vi "Run.vi"(7 "Team Index":i32, 8 "Column":i32, 9 "Row":i32, 10 "View":i32[](array[numeric]) caption="View (Team Index, -1: empty)", 11 "Runner in":refnum<class "Finish.lvclass">) -> (0 "Replicated":refnum<class "Square.lvclass">, 1 "Direction":T1, 2 "Action":T2, 3 "Square Out":refnum<class "Square.lvclass">)   [LabVIEW 2015, in "Finish.lvclass"]
uses:
  Finish.lvclass
  Square/Square.lvclass
  Type Defs/Action Enum.ctl
  Type Defs/Direction Enum.ctl
  Common/Attack Options.ctl
  Common/Find Enemy.vi
  Common/Reverse Direction.vi
  Common/Common.lvlib
  Type Defs/SB Type Defs.lvlib
panel:
  # "NW\nN\nNE\nE\nSE\nS\nSW\nW"
  # "NOTICE - YOU MUST NOT REMOVE THIS NOTICE. PER THE FOLLOWING LICENSE, YOU MAY REPRODUCE THIS SOFTWARE PROVIDED YOU FOLLOW THE TERMS\nOF THE LICENSE.\n\n---BEGIN BSD LICENSE (http://opensource.org/licenses/BSD-2-Clause)---\nCopyright (c) 2015, Endigit, Inc. <robert@endigit.com>\nAll rights reserved.\n\nRedistribution and use in source and binary forms, with or without modification, are permitted provided that the following conditions are met:\n\n1. Redistributions of source code must retain the above copyright notice, this list of conditions and the following disclaimer.\n\n2. Redistributions in binary form must reproduce the above copyright notice, this list of conditions and the following disclaimer in the documentation and/or other \nmaterials provided with the distribution.\n\nTHIS SOFTWARE IS PROVIDED BY THE COPYRIGHT HOLDERS AND CONTRIBUTORS \"AS IS\" AND ANY EXPRESS OR IMPLIED WARRANTIES, INCLUDING, BUT NOT \nLIMITED TO, THE IMPLIED WARRANTIES OF MERCHANTABILITY AND FITNESS FOR A PARTICULAR PURPOSE ARE DISCLAIMED. IN NO EVENT SHALL THE COPYRIGHT \nHOLDER OR CONTRIBUTORS BE LIABLE FOR ANY DIRECT, INDIRECT, INCIDENTAL, SPECIAL, EXEMPLARY, OR CONSEQUENTIAL DAMAGES (INCLUDING, BUT NOT \nLIMITED TO, PROCUREMENT OF SUBSTITUTE GOODS OR SERVICES; LOSS OF USE, DATA, OR PROFITS; OR BUSINESS INTERRUPTION) HOWEVER CAUSED AND ON \nANY THEORY OF LIABILITY, WHETHER IN CONTRACT, STRICT LIABILITY, OR TORT (INCLUDING NEGLIGENCE OR OTHERWISE) ARISING IN ANY WAY OUT OF THE USE \nOF THIS SOFTWARE, EVEN IF ADVISED OF THE POSSIBILITY OF SUCH DAMAGE.\n---END BSD LICENSE---"
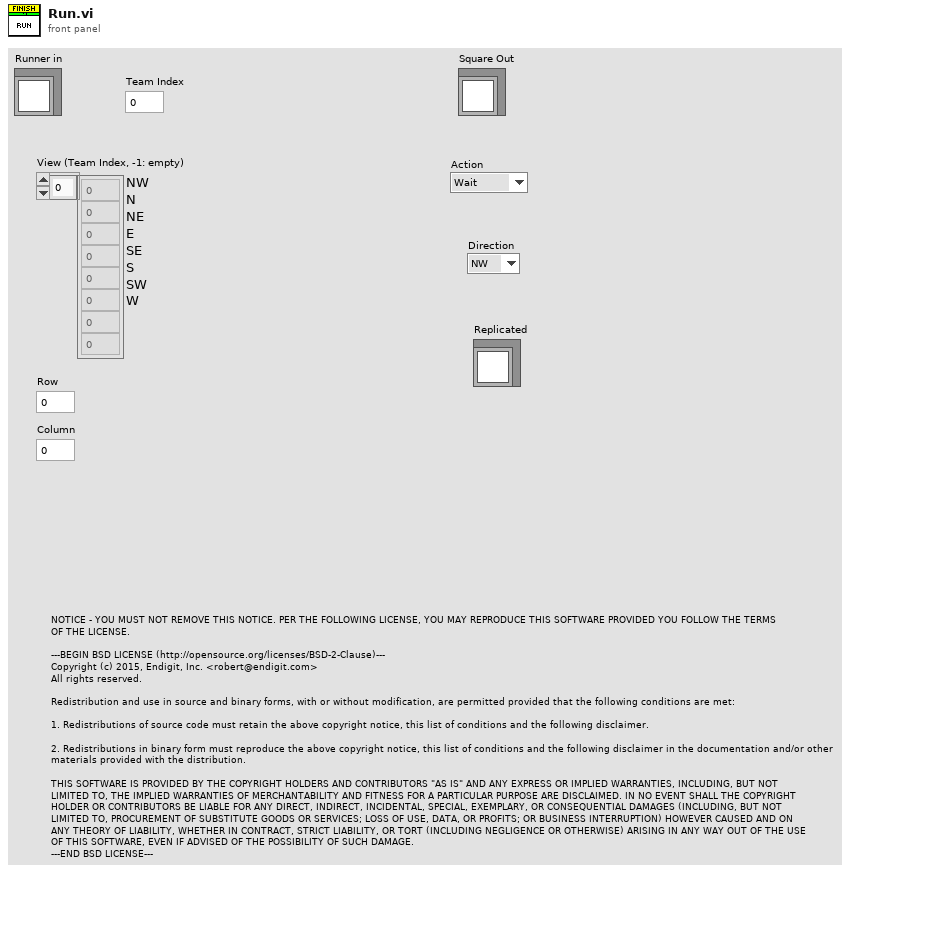
[diagram p1: front panel]
types:
  T1 = typedef "SB Type Defs.lvlib/Direction Enum.ctl" = enum16{"NW", "N", "NE", "E", "SE", "S", "SW", "W"}
  T2 = typedef "SB Type Defs.lvlib/Action Enum.ctl" = enum16{"Wait", "Move", "Attack", "Replicate"}
  T3 = typedef "Common.lvlib/Attack Options.ctl" = enum16{"Attack", "Run", "Distract"}
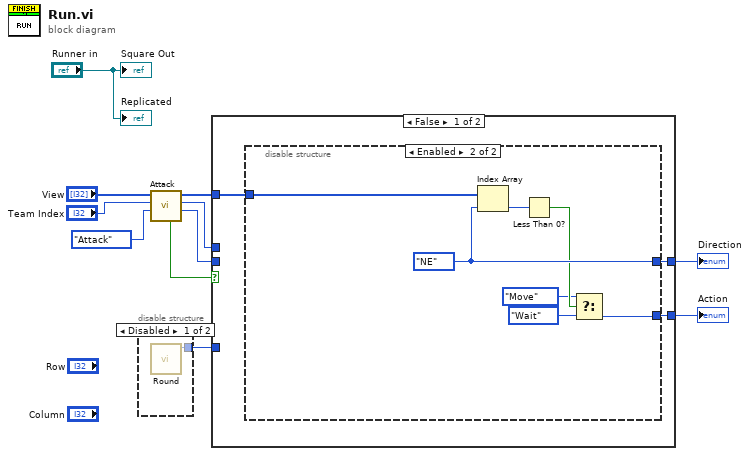
[diagram p0: block diagram]
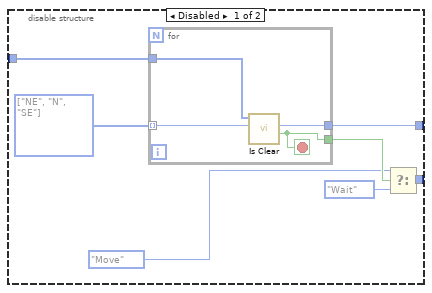
[diagram p3: hidden frame]
diagram:
  n1 = disable-structure shown="Disabled" {
    disable-tunnel: [w12 _] -> w3
    frame Disabled {
      n2 = call "Round.vi"() -> ("Round"=w12:i32)  [unwired: 11 in]
    }
    frame Enabled {
    }
  }
  n3 = call "Attack.vi"("Attack?"=Attack_Options."Attack" ("Attack"), "Team Index"="Team Index", "View"="View") -> ("Direction"=w10:i32, "Action"=w8:T2, "View"=w6:i32[], "Enemy Found?"=w11:bool)  [unwired: 3 in, 2 out]
  n4 = case shown="False" w11 {
    tunnel: w10 -> [_ w35]
    tunnel: [w13 w35] -> w9
    tunnel: w8 -> [_ w34]
    tunnel: [w15 w34] -> w7
    tunnel: w6 -> [w14 _]
    tunnel: w3 -> [_ _]
    frame False {
      n5 = disable-structure shown="Enabled" {
        disable-tunnel: [w22 w29] -> w15
        disable-tunnel: w14 -> [w19 w32]
        disable-tunnel: [w18 w31] -> w13
        frame Disabled {
          w16 = T1[] [enum."NE", enum."N", enum."SE"] items=["NW", "N", "NE", "E", "SE", "S", "SW", "W"]
          n6 = for {
            tunnel: [w25] -> w21
            tunnel: w16 -> [w23] mode=indexing
            tunnel: w19 -> [w26]
            tunnel: [w24] -> w18
            stop <- w25 stop-if-true
            n7 = call "Is Clear.vi"("Direction"=w23, "Maze"=w26) -> ("Can Move?"=w25:bool, "Direction Out"=w24:T1)  [unwired: 7 in, 1 out]
          }
          n8 = Select(t=Action_Enum."Move" ("Action"), s=w21, f=Action_Enum."Wait" ("Action")) -> (s? t:f=w22:T2)
        }
        frame Enabled {
          w31 = Direction_Enum."NE" ("Direction Out")
          n9 = Index Array(array=w32, index=w31) -> (element=w30:i32)
          n10 = Less Than 0?(x=w30) -> (x < 0?=w28:bool)
          n11 = Select(t=Action_Enum."Move", s=w28, f=Action_Enum."Wait" ("Action")) -> (s? t:f=w29:T2)
        }
      }
    }
    frame True {
    }
  }
  "Action" <- w7
  "Direction" <- w9
  "Square Out" <- "Runner in"
  "Replicated" <- "Runner in"
